vi "Internal Message Loop.vi"(8 "error in (no error)":errorcluster, 11 "WAMP Client in":refnum<class "WAMP Client.lvclass">) -> (0 "error out":errorcluster, 3 "WAMP Client out":refnum<class "WAMP Client.lvclass">)   [LabVIEW 2021, in "wamplv.lvlib" / "WAMP Client.lvclass"]
uses:
  WAMP Client.lvclass
  WAMP Client.lvclass/WAMP Client.ctl
  TypeDef/EVENT payload.ctl
  TypeDef/Subscribe Result.ctl
  TypeDef/SUBSCRIBE Request Data.ctl
  TypeDef/WAMP Message Codes.ctl
  TypeDef/WAMP Received Message.ctl
  TypeDef/UNSUBSCRIBE Result.ctl
  TypeDef/UNSUBSCRIBE Request Data.ctl
  TypeDef/PUBLISH Request Data.ctl
  TypeDef/SUBSCRIBE Requests Map.ctl
  TypeDef/Subscription Details.ctl
  TypeDef/Subscriptions Map.ctl
  TypeDef/Unsubscribe Requests Map.ctl
  TypeDef/Publish Requests Map.ctl
  TypeDef/Termination Reason Enum.ctl
  TypeDef/GOODBYE Request Data.ctl
  API/TypeDefs/RESULT payload.ctl
  TypeDef/CALL Request Data.ctl
  API/TypeDefs/WAMP error.ctl
  TypeDef/Success or error.ctl
  TypeDef/REGISTER Request Data.ctl
  TypeDef/Message Loop Shift Reg Data.ctl
  TypeDef/Endpoint Data.ctl
  TypeDef/CALL Request Map.ctl
  API/TypeDefs/Combined error.ctl
  TypeDef/Unregister request.ctl
  TypeDef/Unregister requests map.ctl
  TypeDef/PUBLISH result.ctl
  0ad20a80-b884-3f82-8ee8-d8e935c3ee3f.vi
  08e67e80-cc16-3fac-40e3-ebe0e858da3f.vi
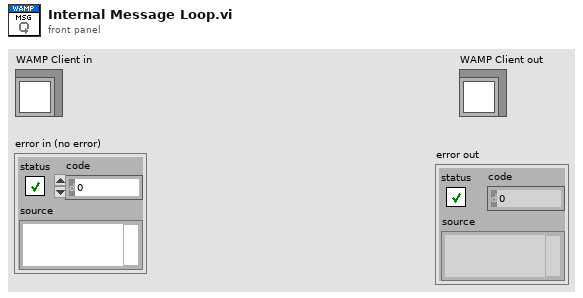
[diagram p1: front panel]
types:
  T1 = typedef "wamplv.lvlib/WAMP Client.lvclass/Message Loop Shift Reg Data.ctl" = cluster{"Last Request ID":u64, "Register Requests":map{u64, T2}, "Publish Requests":T3, "Endpoints Map":map{u64, T5}, "Call Requests":T6, "Subscription Requests":T8, "Subscriptions":T10, "Unsubscribe Requests":T12, "Random Request IDs":u64[], "Unregister requests map":T14}
  T2 = typedef "wamplv.lvlib/WAMP Client.lvclass/REGISTER Request Data.ctl" = cluster{"Procedure URI":string, "Options":string, "REGISTER result notifier":refnum<notifier>}
  T3 = typedef "wamplv.lvlib/WAMP Client.lvclass/Publish Requests Map.ctl" = map{u64, T4}
  T4 = typedef "wamplv.lvlib/WAMP Client.lvclass/PUBLISH Request Data.ctl" = cluster{"Topic URI":string, "Arguments":string, "ArgumentsKw":string, "Request Acknowledgement":bool, "Options":string, "Publish result notifier":refnum<notifier>}
  T5 = typedef "wamplv.lvlib/WAMP Client.lvclass/Endpoint Data.ctl" = cluster{"Procedure URI":string}
  T6 = typedef "wamplv.lvlib/WAMP Client.lvclass/CALL Request Map.ctl" = map{u64, T7}
  T7 = typedef "wamplv.lvlib/WAMP Client.lvclass/CALL Request Data.ctl" = cluster{"Topic URI":string, "Arguments":string, "ArgumentsKw":string, "Options":string, "Call result":refnum<notifier>}
  T8 = typedef "wamplv.lvlib/WAMP Client.lvclass/SUBSCRIBE Requests Map.ctl" = map{u64, T9}
  T9 = typedef "wamplv.lvlib/WAMP Client.lvclass/SUBSCRIBE Request Data.ctl" = cluster{"Topic":string, "Subscribe result notifer":refnum<notifier>}
  T10 = typedef "wamplv.lvlib/WAMP Client.lvclass/Subscriptions Map.ctl" = map{u64, T11}
  T11 = typedef "wamplv.lvlib/WAMP Client.lvclass/Subscription Details.ctl" = cluster{"Subscription ID":u64, "Topic":string, "Publication Received Event":refnum<user-event>}
  T12 = typedef "wamplv.lvlib/WAMP Client.lvclass/Unsubscribe Requests Map.ctl" = map{u64, T13}
  T13 = typedef "wamplv.lvlib/WAMP Client.lvclass/UNSUBSCRIBE Request Data.ctl" = cluster{"Topic":string, "Unsubscrube result notifier":refnum<notifier>}
  T14 = typedef "wamplv.lvlib/WAMP Client.lvclass/Unregister requests map.ctl" = map{u64, T15}
  T15 = typedef "wamplv.lvlib/WAMP Client.lvclass/Unregister request.ctl" = cluster{"URI":string, "Unregister result notifier":refnum<notifier>}
  T16 = typedef "wamplv.lvlib/WAMP Client.lvclass/Termination Reason Enum.ctl" = enum16{"Goodbye Received", "Abort Received", "Send Goodbye", "Send Abort", "Read Loop Failure", "Write Loop Failure", "Message Loop Failure"}
  T17 = typedef "wamplv.lvlib/WAMP Client.lvclass/WAMP Received Message.ctl" = cluster{"Message JSON":string[], "Message Codes":T18}
  T18 = typedef "wamplv.lvlib/WAMP Client.lvclass/WAMP Message Codes.ctl" = u16
  T19 = typedef "wamplv.lvlib/WAMP Client.lvclass/GOODBYE Request Data.ctl" = cluster{"Error URI":string, "Message":string}
  T20 = typedef "wamplv.lvlib/WAMP Client.lvclass/Internal Message.ctl" = cluster{"Internal Message Type":T21, "Variant":variant}
  T21 = typedef "wamplv.lvlib/WAMP Client.lvclass/Internal Message Type.ctl" = enum16{"Subscribe", "Handle Subscribed", "Handle Event", "Unsubscribe", "Handle Unsubscribed", "Publish", "Handled Published", "Goodbye", "Handle Goodbye", "Call", "Handle Result", "Register", "Handle Registered", "Unregister", "Handle Unregistered", "Handle Invocation", "Yield", "Error"}
  T22 = typedef "wamplv.lvlib/WAMP Client.lvclass/YIELD request data.ctl" = cluster{"Invocation Request ID":u64, "Arguments":string, "ArgumentsKw":string, "Options":string}
  T23 = typedef "wamplv.lvlib/WAMP Client.lvclass/Error Request.ctl" = cluster{"WAMP Error":T24, "Message Type":T18, "Request ID":u64}
  T24 = typedef "wamplv.lvlib/WAMP Client.lvclass/WAMP error.ctl" = cluster{"Details":string, "ArgumentKw Payload":string, "Error?":bool, "Error URI":string, "Arguments Payload":string}
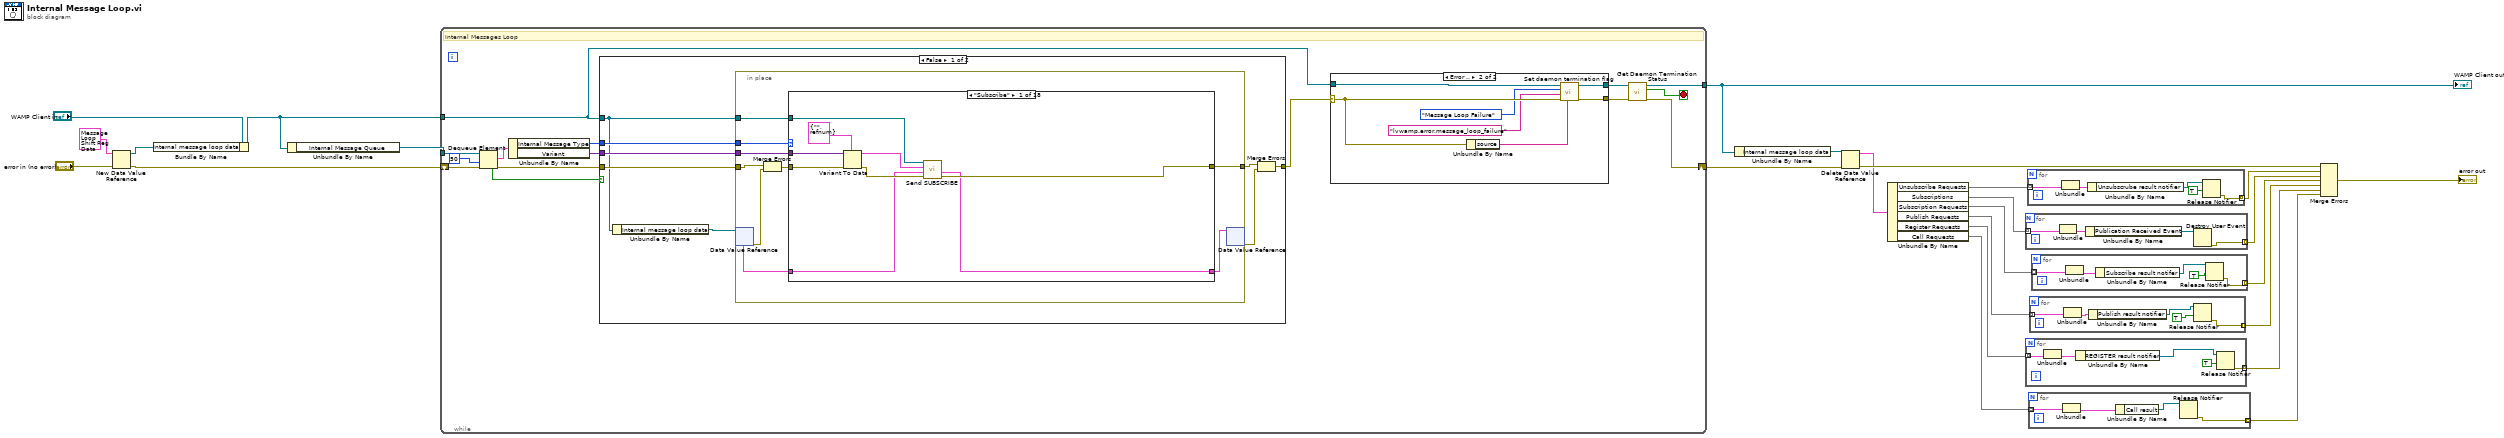
[diagram p0: block diagram]
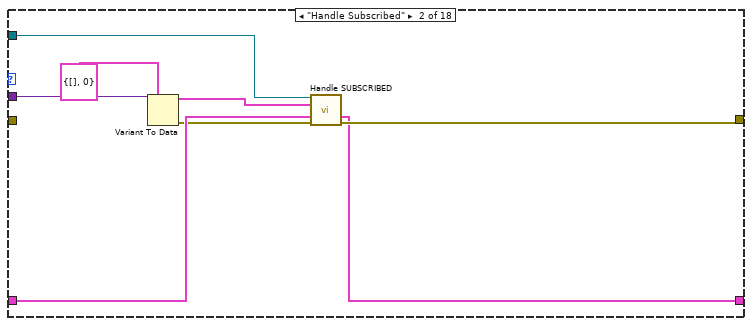
[diagram p3: hidden frame]
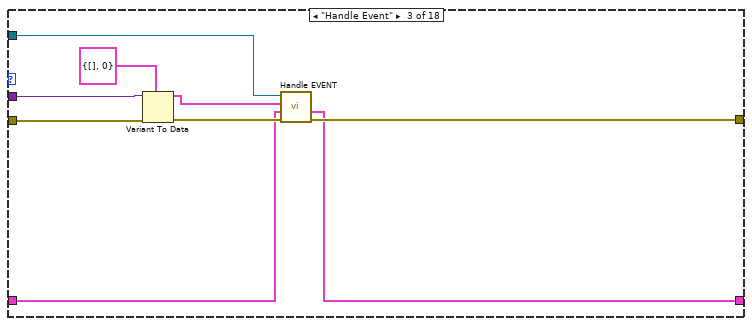
[diagram p4: hidden frame]
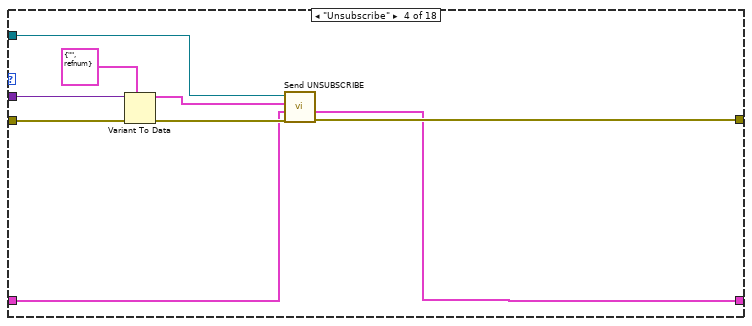
[diagram p5: hidden frame]
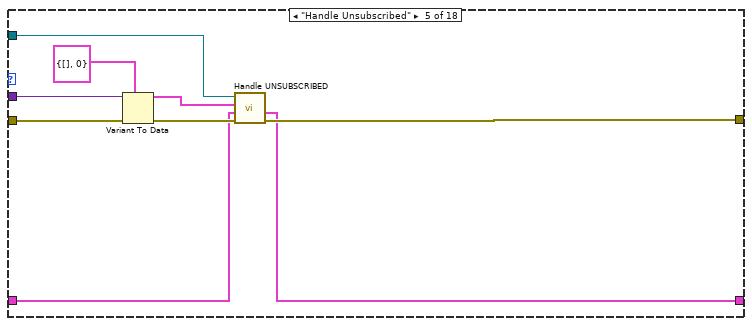
[diagram p6: hidden frame]
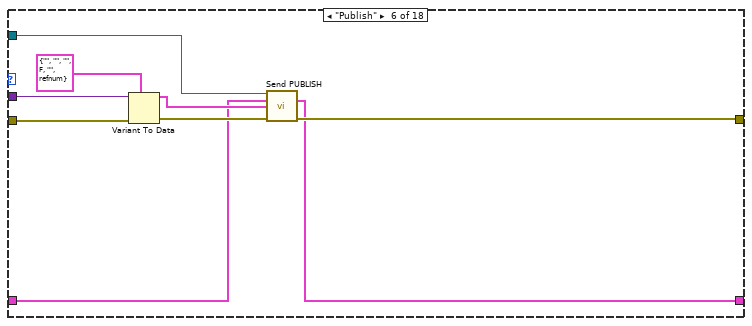
[diagram p7: hidden frame]
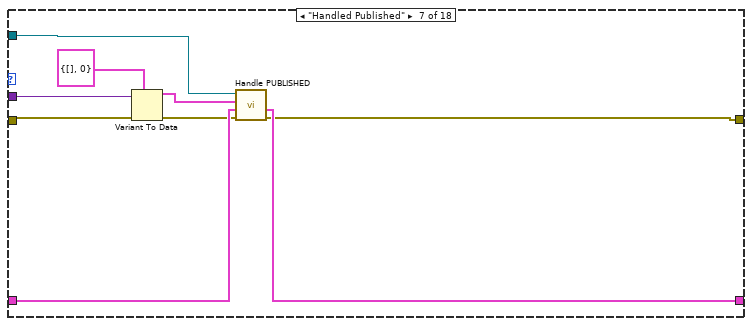
[diagram p8: hidden frame]
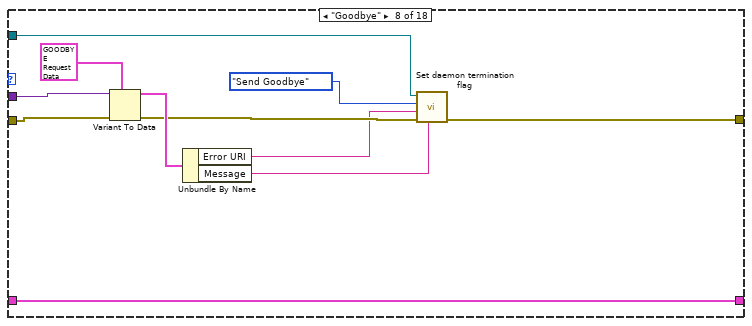
[diagram p9: hidden frame]
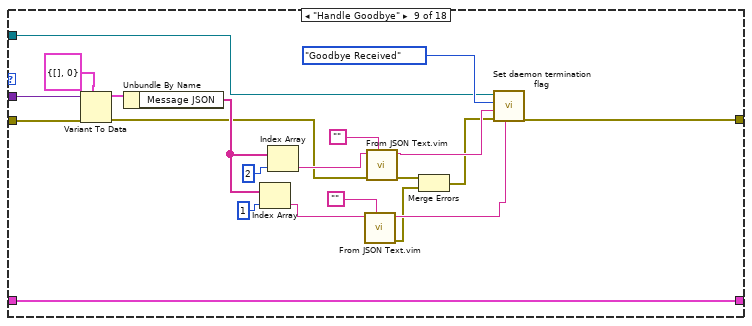
[diagram p10: hidden frame]
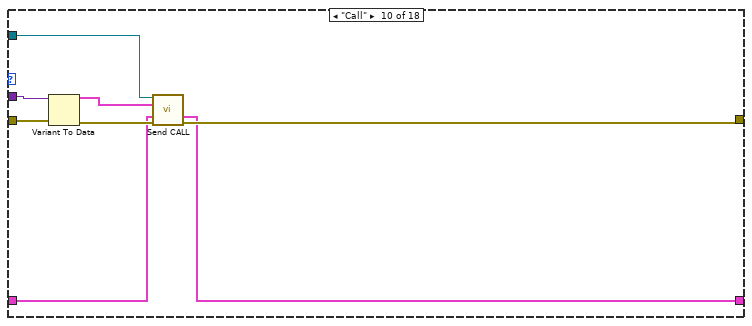
[diagram p11: hidden frame]
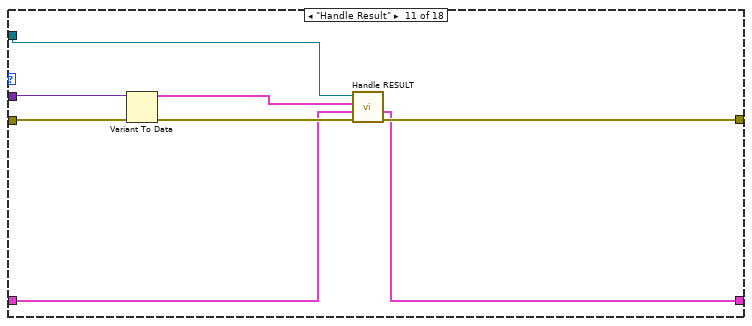
[diagram p12: hidden frame]
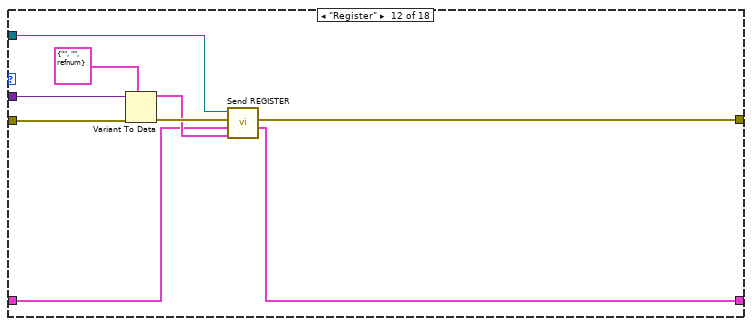
[diagram p13: hidden frame]
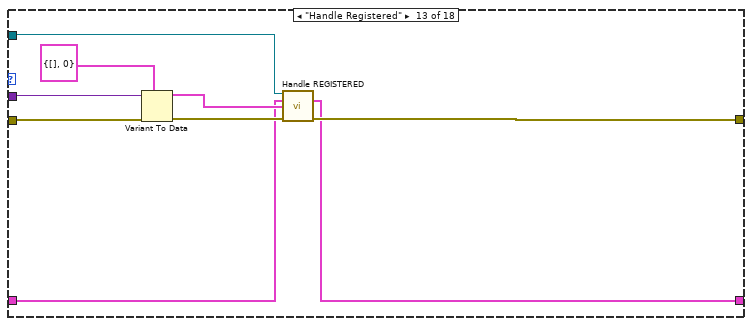
[diagram p14: hidden frame]
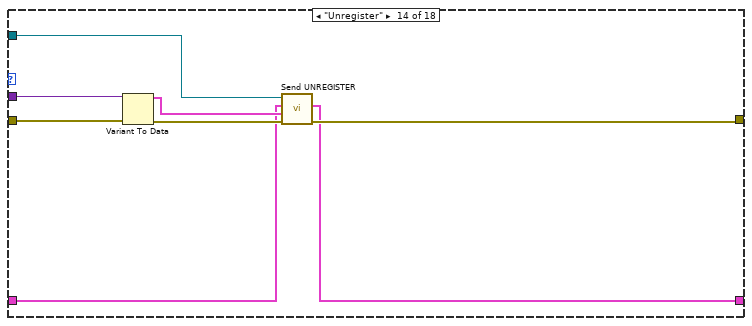
[diagram p15: hidden frame]
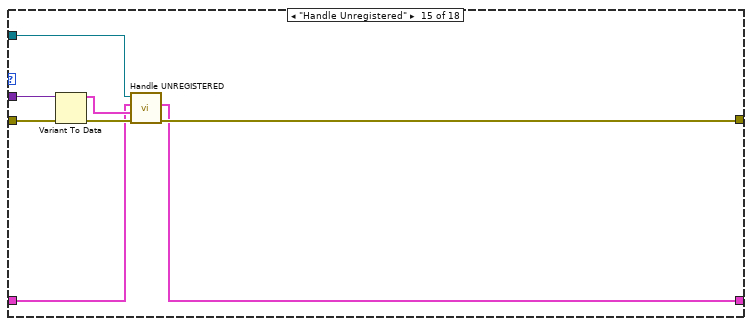
[diagram p16: hidden frame]
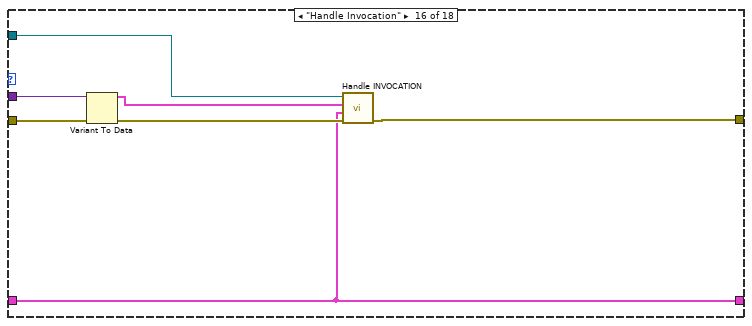
[diagram p17: hidden frame]
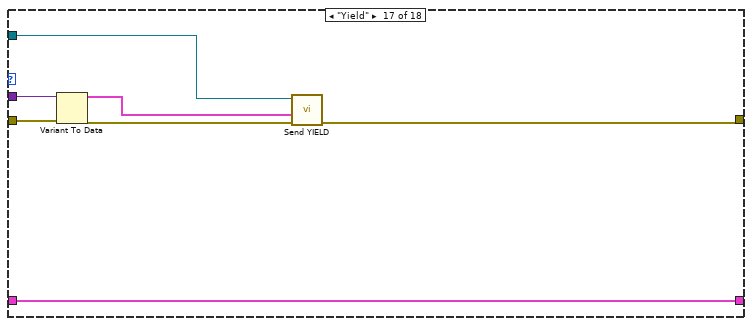
[diagram p18: hidden frame]
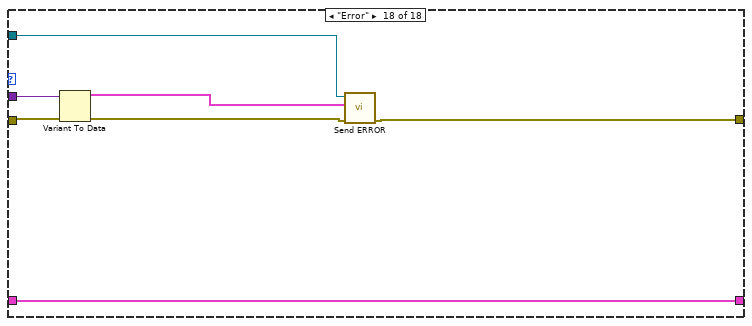
[diagram p19: hidden frame]
diagram:
  n1 = New Data Value Reference(data value=T1 {"Last Request ID"=0, "Register Requests"={}, "Publish Requests"={}, "Endpoints Map"={}, "Call Requests"={}, "Subscription Requests"={}, "Subscriptions"={}, "Unsubscribe Requests"={}, "Random Request IDs"=[], "Unregister requests map"={}} ("Message Loop Shift Register Data"), error in="error in (no error)") -> (data value reference=w10:refnum<data-value>, error out=w8:errorcluster)
  n2 = Bundle By Name(cluster="WAMP Client in", "Internal message loop data"=w10) -> (w7:refnum<class "WAMP Client.lvclass">)
  n3 = Unbundle By Name(w7) -> ("Internal Message Queue"=w25:refnum<queue>)
  n4 = while {
    tunnel: w25 -> [w39]
    tunnel: w7 -> [w27]
    shift-right: [w29] -> w3
    shift-left: w8 -> [w34]
    tunnel: [w26] -> w6
    stop <- w28 stop-if-true
    # "Internal Messages Loop"
    n5 = Dequeue Element(queue=w39, timeout in ms (-1)=50, error in (no error)=w34) -> (element=w38:T20, timed out?=w35:bool, error out=w33:errorcluster)  [unwired: 1 out]
    n6 = Unbundle By Name(w38) -> ("Internal Message Type"=w37:T21, "Variant"=w36:variant)
    n7 = case shown="False" w35 {
      tunnel: w37 -> [w57 _]
      tunnel: w36 -> [w56 _]
      tunnel: w27 -> [w54 _]
      tunnel: w33 -> [w55 w232]
      tunnel: [w52 w232] -> w32
      frame False {
        n8 = Unbundle By Name(w54) -> ("Internal message loop data"=w53:refnum<data-value>)
        n9 = in-place {
          in-place-border: w57 -> [w66]
          in-place-border: w56 -> [w65]
          in-place-border: w54 -> [w64]
          in-place-border: w55 -> [w61]
          in-place-border: [w63] -> w51
          n10 = in-place-dvr #1(w53) -> (w59:T1, w60:errorcluster)
          n11 = Merge Errors(w61, w60) -> (w62:errorcluster)
          n12 = case shown="\"Subscribe\"" w66 {
            tunnel: w65 -> [w75 w82 w91 w101 w110 w119 w127 w139 w158 w168 w175 w184 w194 w202 w208 w216 w224 w227]
            tunnel: w64 -> [w73 w83 w92 w100 w108 w114 w124 w133 w151 w166 w176 w179 w190 w198 w206 w217 w220 w230]
            tunnel: w62 -> [w70 _ w89 w97 w106 w116 w125 w137 w159 w167 w174 w182 w193 w201 w210 w215 w223 w228]
            tunnel: [w69 w77 w88 w95 w103 w112 w121 w135 w160 w162 w172 w178 w188 w197 w204 w213 w219 w231] -> w63
            tunnel: w59 -> [w68 w80 w85 w94 w104 w113 w123 w129 w150 w163 w170 w180 w187 w196 w205 w211 w218 w225]
            tunnel: [w67 w76 w84 w93 w102 w111 w122 w129 w150 w161 w169 w177 w186 w195 w203 w211 w218 w225] -> w58
            frame "Subscribe" {
              n13 = Variant To Data(error in=w70, type=T9 {"Topic"="", "Subscribe result notifer"=refnum} ("Cluster"), Variant=w75) -> (data=w72:T9, error out=w71:errorcluster)
              n14 = call-dynamic "Send SUBSCRIBE.vi"("error in (no error)"=w71, "Message Loop Data (in)"=w68, "Subscription Request"=w72, "WAMP Client in"=w73) -> ("error out"=w69:errorcluster, "Message Loop Data (out)"=w67:T1)  [unwired: 5 in, 1 out]
            }
            frame "Handle Subscribed" {
              n15 = Variant To Data(type=T17 {"Message JSON"=[], "Message Codes"=0} ("Cluster"), Variant=w82) -> (data=w79:T17, error out=w78:errorcluster)  [unwired: 1 in]
              n16 = call-dynamic "Handle SUBSCRIBED.vi"("reference"=w83, "WAMP Message"=w79, "Message Loop data (in)"=w80, "error in (no error)"=w78) -> ("Message Loop Data (out)"=w76:T1, "error out"=w77:errorcluster)  [unwired: 9 in, 1 out]
            }
            frame "Handle Event" {
              n17 = Variant To Data(error in=w89, type=T17 {"Message JSON"=[], "Message Codes"=0} ("Cluster"), Variant=w91) -> (data=w86:T17, error out=w87:errorcluster)
              n18 = call-dynamic "Handle EVENT.vi"("error in (no error)"=w87, "Message Loop Data (in)"=w85, "Cluster"=w86, "reference"=w92) -> ("error out"=w88:errorcluster, "Message Loop Data (out)"=w84:T1)  [unwired: 5 in, 1 out]
            }
            frame "Unsubscribe" {
              n19 = Variant To Data(error in=w97, type=T13 {"Topic"="", "Unsubscrube result notifier"=refnum} ("Cluster"), Variant=w101) -> (data=w99:T13, error out=w96:errorcluster)
              n20 = call-dynamic "Send UNSUBSCRIBE.vi"("error in (no error)"=w96, "Message loop data (in)"=w94, "Unsubscribe Request Data"=w99, "WAMP Client in"=w100) -> ("error out"=w95:errorcluster, "Message loop data (out)"=w93:T1)  [unwired: 5 in, 1 out]
            }
            frame "Handle Unsubscribed" {
              n21 = Variant To Data(error in=w106, type=T17 {"Message JSON"=[], "Message Codes"=0} ("Cluster"), Variant=w110) -> (data=w107:T17, error out=w105:errorcluster)
              n22 = call-dynamic "Handle UNSUBSCRIBED.vi"("error in (no error)"=w105, "Message Loop data (in)"=w104, "WAMP Message"=w107, "reference"=w108) -> ("error out"=w103:errorcluster, "Message Loop Data (Out)"=w102:T1)  [unwired: 5 in, 1 out]
            }
            frame "Publish" {
              n23 = Variant To Data(error in=w116, type=T4 {"Topic URI"="", "Arguments"="", "ArgumentsKw"="", "Request Acknowledgement"=FALSE, "Options"="", "Publish result notifier"=refnum} ("Cluster"), Variant=w119) -> (data=w117:T4, error out=w115:errorcluster)
              n24 = call-dynamic "Send PUBLISH.vi"("WAMP Client in"=w114, "Message Loop Shift Register Data (In)"=w113, "Publish Request Data"=w117, "error in (no error)"=w115) -> ("Message Loop Shift Register Data (Out)"=w111:T1, "error out"=w112:errorcluster)  [unwired: 9 in, 1 out]
            }
            frame "Handled Published" {
              n25 = Variant To Data(error in=w125, type=T17 {"Message JSON"=[], "Message Codes"=0} ("Cluster"), Variant=w127) -> (data=w126:T17, error out=w120:errorcluster)
              n26 = call-dynamic "Handle PUBLISHED.vi"("error in (no error)"=w120, "Message Loop data (in)"=w123, "WAMP Message"=w126, "reference"=w124) -> ("error out"=w121:errorcluster, "Message Loop data (out)"=w122:T1)  [unwired: 5 in, 1 out]
            }
            frame "Goodbye" {
              n27 = Variant To Data(error in=w137, type=T19 {"Error URI"="wamp.error.protocol_violation", "Message"="wamp.close.shut_down"} ("Goodbye Request"), Variant=w139) -> (data=w136:T19, error out=w134:errorcluster)
              n28 = Unbundle By Name(w136) -> ("Error URI"=w131:string, "Message"=w130:string)
              n29 = call "Set daemon termination flag.vi"("Message"=w130, "error in (no error)"=w134, "Reason URI"=w131, "Reason"=Termination_Reason_Enum."Send Goodbye" ("Termination Reason"), "WAMP Client (in)"=w133) -> ("error out"=w135:errorcluster)  [unwired: 5 in, 1 out]
            }
            frame "Handle Goodbye" {
              n30 = Variant To Data(error in=w159, type=T17 {"Message JSON"=[], "Message Codes"=0} ("Cluster"), Variant=w158) -> (data=w156:T17, error out=w143:errorcluster)
              n31 = Unbundle By Name(w156) -> ("Message JSON"=w153:string[])
              n32 = Index Array(array=w153, index=1) -> (element=w145:string)
              n33 = Index Array(array=w153, index=2) -> (element=w149:string)
              n34 = call "From JSON Text.vim"("Data Type and Default Value"="", "JSON"=w145) -> ("error out"=w140:errorcluster, "Data out"=w146:string)  [unwired: 8 in]
              n35 = call "From JSON Text.vim"("Data Type and Default Value"="", "error in (no error)"=w143, "JSON"=w149) -> ("error out"=w141:errorcluster, "Data out"=w147:string)  [unwired: 7 in]
              n36 = Merge Errors(w141, w140) -> (w142:errorcluster)
              n37 = call "Set daemon termination flag.vi"("Message"=w146, "error in (no error)"=w142, "Reason URI"=w147, "Reason"=Termination_Reason_Enum."Goodbye Received" ("Termination Reason"), "WAMP Client (in)"=w151) -> ("error out"=w160:errorcluster)  [unwired: 5 in, 1 out]
            }
            frame "Call" {
              n38 = Variant To Data(error in=w167, Variant=w168) -> (data=w164:T7, error out=w165:errorcluster)  [unwired: 1 in]
              n39 = call-dynamic "Send CALL.vi"("WAMP Client in"=w166, "Call Request"=w164, "Message Loop Shift Register Data"=w163, "error in (no error)"=w165) -> ("Message Loop Shift Register Data (out)"=w161:T1, "error out"=w162:errorcluster)  [unwired: 9 in, 1 out]
            }
            frame "Handle Result" {
              n40 = Variant To Data(error in=w174, Variant=w175) -> (data=w173:T17, error out=w171:errorcluster)  [unwired: 1 in]
              n41 = call-dynamic "Handle RESULT.vi"("error in (no error)"=w171, "Message Loop Shift Register Data"=w170, "WAMP Message"=w173, "reference"=w176) -> ("error out"=w172:errorcluster, "Message Loop Shift Register Data (out)"=w169:T1)  [unwired: 5 in, 1 out]
            }
            frame "Register" {
              n42 = Variant To Data(error in=w182, type=T2 {"Procedure URI"="", "Options"="", "REGISTER result notifier"=refnum} ("REGISTER request data"), Variant=w184) -> (data=w181:T2, error out=w183:errorcluster)
              n43 = call-dynamic "Send REGISTER.vi"("REGISTER request data"=w181, "Message Loop Shift Register Data"=w180, "error in (no error)"=w183, "WAMP Client in"=w179) -> ("Message Loop Shift Register Data"=w177:T1, "error out"=w178:errorcluster)  [unwired: 5 in, 1 out]
            }
            frame "Handle Registered" {
              n44 = Variant To Data(error in=w193, type=T17 {"Message JSON"=[], "Message Codes"=0} ("Cluster"), Variant=w194) -> (data=w192:T17, error out=w189:errorcluster)
              n45 = call-dynamic "Handle REGISTERED.vi"("reference"=w190, "Message Loop Shift Register Data"=w187, "WAMP Message"=w192, "error in (no error)"=w189) -> ("output cluster"=w186:T1, "error out"=w188:errorcluster)  [unwired: 9 in, 1 out]
            }
            frame "Unregister" {
              n46 = Variant To Data(error in=w201, Variant=w202) -> (data=w200:T15, error out=w199:errorcluster)  [unwired: 1 in]
              n47 = call-dynamic "Send UNREGISTER.vi"("error in (no error)"=w199, "Unregister Request"=w200, "Message loop data (in)"=w196, "WAMP Client in"=w198) -> ("error out"=w197:errorcluster, "Message loop data (out)"=w195:T1)  [unwired: 5 in, 1 out]
            }
            frame "Handle Unregistered" {
              n48 = Variant To Data(error in=w210, Variant=w208) -> (data=w207:T17, error out=w209:errorcluster)  [unwired: 1 in]
              n49 = call-dynamic "Handle UNREGISTERED.vi"("error in (no error)"=w209, "WAMP Message"=w207, "Message loop data (in)"=w205, "reference"=w206) -> ("error out"=w204:errorcluster, "Message Loop Data (Out)"=w203:T1)  [unwired: 5 in, 1 out]
            }
            frame "Handle Invocation" {
              n50 = Variant To Data(error in=w215, Variant=w216) -> (data=w212:T17, error out=w214:errorcluster)  [unwired: 1 in]
              n51 = call-dynamic "Handle INVOCATION.vi"("error in (no error)"=w214, "Message Loop Shift Register Data"=w211, "Cluster"=w212, "reference"=w217) -> ("error out"=w213:errorcluster)  [unwired: 6 in, 1 out]
            }
            frame "Yield" {
              n52 = Variant To Data(error in=w223, Variant=w224) -> (data=w222:T22, error out=w221:errorcluster)  [unwired: 1 in]
              n53 = call-dynamic "Send YIELD.vi"("error in (no error)"=w221, "Yield request"=w222, "WAMP Client in"=w220) -> ("error out"=w219:errorcluster)  [unwired: 7 in, 1 out]
            }
            frame "Error" {
              n54 = Variant To Data(error in=w228, Variant=w227) -> (data=w226:T23, error out=w229:errorcluster)  [unwired: 1 in]
              n55 = call-dynamic "Send ERROR.vi"("error in (no error)"=w229, "Error Request"=w226, "WAMP Client in"=w230) -> ("error out"=w231:errorcluster)  [unwired: 7 in, 1 out]
            }
          }
          n56 = in-place-dvr #1(w58) -> (w50:errorcluster)  [unwired: 1 out]
        }
        n57 = Merge Errors(w51, w50) -> (w52:errorcluster)
      }
      frame True {
        # "Time out, no internal messages"
      }
    }
    n58 = case shown="Error .." w32 {
      selector: w32 -> [w42 w48]
      tunnel: [w42 w49] -> w31
      tunnel: [w41 w47] -> w30
      tunnel: w27 -> [w41 w46]
      frame No Error {
      }
      frame Error {
        n59 = Unbundle By Name(w48) -> ("source"=w43:string)
        n60 = call "Set daemon termination flag.vi"("Message"=w43, "error in (no error)"=w48, "Reason URI"="lvwamp.error.message_loop_failure" ("Error URI"), "Reason"=Termination_Reason_Enum."Message Loop Failure" ("Termination Reason"), "WAMP Client (in)"=w46) -> ("error out"=w49:errorcluster, "WAMP Client (out)"=w47:refnum<class "WAMP Client.lvclass">)  [unwired: 5 in]
      }
    }
    n61 = call "Get Daemon Termination Status.vi"("error in (no error)"=w31, "WAMP Client in"=w30) -> ("error out"=w29:errorcluster, "Terminate?"=w28:bool, "WAMP Client out"=w26:refnum<class "WAMP Client.lvclass">)  [unwired: 6 in, 1 out]
  }
  "WAMP Client out" <- w6
  n62 = Unbundle By Name(w6) -> ("Internal message loop data"=w5:refnum<data-value>)
  n63 = Delete Data Value Reference(data value reference=w5, error in=w3) -> (data value=w1:T1, error out=w4:errorcluster)
  n64 = Unbundle By Name(w1) -> ("Unsubscribe Requests"=w19:T12, "Subscriptions"=w20:T10, "Subscription Requests"=w21:T8, "Publish Requests"=w24:T3, "Register Requests"=w23:map{u64, T2}, "Call Requests"=w22:T6)
  n65 = for {
    tunnel: w20 -> [w236] mode=indexing
    tunnel: [w233] -> w17 mode=indexing
    n66 = Unbundle(w236) -> (w235:T11)  [unwired: 1 out]
    n67 = Unbundle By Name(w235) -> ("Publication Received Event"=w234:refnum<user-event>)
    n68 = Destroy User Event(user event=w234) -> (error out=w233:errorcluster)  [unwired: 1 in]
  }
  n69 = for {
    tunnel: w23 -> [w241] mode=indexing
    tunnel: [w239] -> w14 mode=indexing
    n70 = Unbundle(w241) -> (w240:T2)  [unwired: 1 out]
    n71 = Unbundle By Name(w240) -> ("REGISTER result notifier"=w238:refnum<notifier>)
    n72 = Release Notifier(notifier=w238, force destroy? (F)=TRUE) -> (error out=w239:errorcluster)  [unwired: 1 in, 2 out]
  }
  n73 = for {
    tunnel: w19 -> [w246] mode=indexing
    tunnel: [w244] -> w18 mode=indexing
    n74 = Unbundle(w246) -> (w245:T13)  [unwired: 1 out]
    n75 = Unbundle By Name(w245) -> ("Unsubscrube result notifier"=w243:refnum<notifier>)
    n76 = Release Notifier(notifier=w243, force destroy? (F)=TRUE) -> (error out=w244:errorcluster)  [unwired: 1 in, 2 out]
  }
  n77 = for {
    tunnel: w22 -> [w250] mode=indexing
    tunnel: [w247] -> w13 mode=indexing
    n78 = Unbundle(w250) -> (w249:T7)  [unwired: 1 out]
    n79 = Unbundle By Name(w249) -> ("Call result"=w248:refnum<notifier>)
    n80 = Release Notifier(notifier=w248) -> (error out=w247:errorcluster)  [unwired: 2 in, 2 out]
  }
  n81 = for {
    tunnel: w24 -> [w255] mode=indexing
    tunnel: [w253] -> w15 mode=indexing
    n82 = Unbundle(w255) -> (w254:T4)  [unwired: 1 out]
    n83 = Unbundle By Name(w254) -> ("Publish result notifier"=w252:refnum<notifier>)
    n84 = Release Notifier(notifier=w252, force destroy? (F)=TRUE) -> (error out=w253:errorcluster)  [unwired: 1 in, 2 out]
  }
  n85 = for {
    tunnel: w21 -> [w260] mode=indexing
    tunnel: [w256] -> w16 mode=indexing
    n86 = Unbundle(w260) -> (w259:T9)  [unwired: 1 out]
    n87 = Unbundle By Name(w259) -> ("Subscribe result notifer"=w258:refnum<notifier>)
    n88 = Release Notifier(notifier=w258, force destroy? (F)=TRUE) -> (error out=w256:errorcluster)  [unwired: 1 in, 2 out]
  }
  n89 = Merge Errors(w4, w18, w17, w16, w15, w14, w13) -> (→"error out":errorcluster)
